vi "available tags menu.vi"(4 "Coords":T2, 5 "parent vi reference":refnum<vi>, 6 "Screen":bool, 8 "error in":errorcluster, 9 "channel to map to":refnum<class "TBM channel.lvclass">, 10 "object ref":T1, 11 "ATM":refnum<user-event>) -> (0 "error out":errorcluster)   [LabVIEW 2013, in "Table Manager.lvlib"]
uses:
  Table Manager.lvlib
  <vilib>/NI/Tag Bus Module Framework/channel/TBM channel.lvclass
  <vilib>/Utility/miscctls.llb/LVPoint32TypeDef.ctl
  <vilib>/NI/DCAF/Tag Editor Core/control module/editor node/channel action event.ctl
  <vilib>/NI/DCAF/Tag Editor Core/control module/editor node/dialog output action.ctl
  <vilib>/NI/Tag Bus/tag/tag descriptor.lvclass
  Table Manager/object ref.ctl
  <vilib>/NI/DCAF/Tag Editor Core/Configuration Editor/Classes/Engine Parent/Engine Parent Editor Node.lvclass
  <vilib>/NI/DCAF/Tag Editor Core/Configuration Editor/Classes/Module editor node/module editor node.lvclass
  <vilib>/NI/DCAF/Tag Editor Core/Configuration Editor/Classes/Engine Parent/read engine configuration.vi
  <vilib>/NI/Module Execution Interface/Engine Configuration/engine configuration.lvclass
  <vilib>/NI/DCAF/Tag Editor Core/control module/editor node/control module editor.lvclass
  Table Manager/Table Manager.lvclass
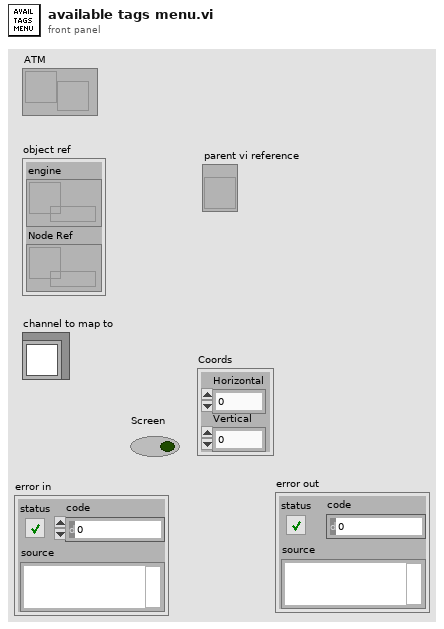
[diagram p1: front panel]
types:
  T1 = typedef "Table Manager.lvlib/Table Manager.lvclass/object ref.ctl" = cluster{"engine":refnum<data-value>, "Node Ref":refnum<data-value>}
  T2 = typedef "LVPoint32TypeDef.ctl" = cluster{"Horizontal":i32, "Vertical":i32}
  T3 = enum32{"Invalid", "Standard", "Closed", "Hidden", "Minimized", "Maximized"}
  T4 = typedef "LVRectTypeDef.ctl" = cluster{"Left":i16, "Top":i16, "Right":i16, "Bottom":i16}
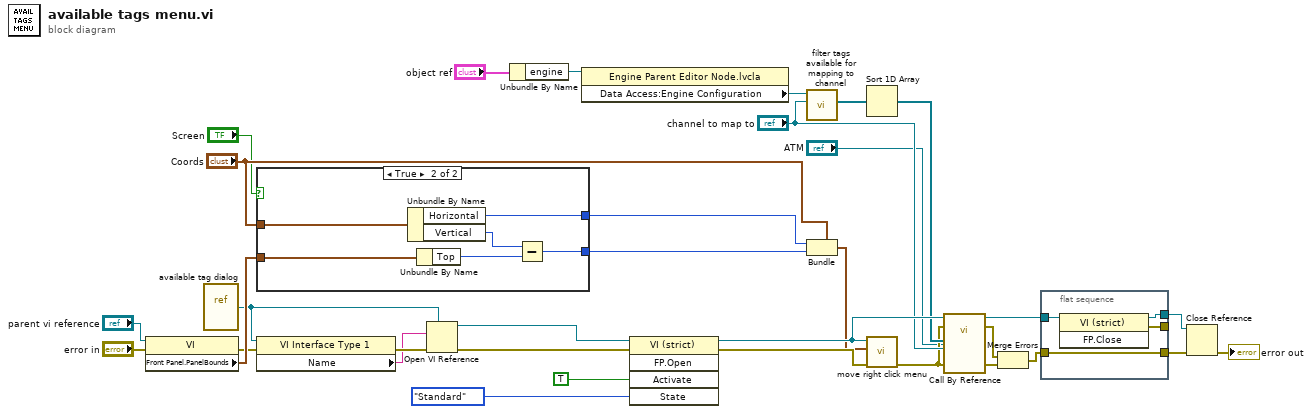
[diagram p0: block diagram]
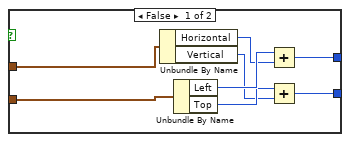
[diagram p2: hidden frame]
diagram:
  n1 = property class="VI"(reference="parent vi reference", error in="error in") -> (error out=w13:errorcluster, "Front Panel.PanelBounds"=w32:T4)  [unwired: 1 out]
  n2 = vi-ref "available tag dialog.vi"() -> (w20:refnum<vi>)
  n3 = case shown="True" "Screen" {
    tunnel: w32 -> [w41 w45]
    tunnel: [w38 w46] -> w31
    tunnel: [w35 w42] -> w30
    tunnel: "Coords" -> [w34 w47]
    frame False {
      n4 = Unbundle By Name(w34) -> ("Horizontal"=w39:i32, "Vertical"=w36:i32)
      n5 = Unbundle By Name(w41) -> ("Left"=w40:i16, "Top"=w37:i16)
      n6 = Add(x=w40, y=w39) -> (x+y=w38:i32)
      n7 = Add(x=w37, y=w36) -> (x+y=w35:i32)
    }
    frame True {
      n8 = Unbundle By Name(w47) -> ("Horizontal"=w46:i32, "Vertical"=w44:i32)
      n9 = Unbundle By Name(w45) -> ("Top"=w43:i16)
      n10 = Subtract(x=w44, y=w43) -> (x-y=w42:i32)
    }
  }
  n11 = property class="VI Interface Type 1"(reference=w20, error in=w13) -> (error out=w27:errorcluster, "Name"=w26:string)  [unwired: 1 out]
  n12 = Open VI Reference(type specifier VI Refnum (for type only)=w20, vi path=w26, error in (no error)=w27) -> (vi reference=w24:refnum<vi>, error out=w25:errorcluster)  [unwired: 3 in]
  n13 = Unbundle By Name("object ref") -> ("engine"=w2:refnum<data-value>)
  n14 = property class="Engine Parent Editor Node.lvcla"(reference=w2) -> ("Data Access:Engine Configuration"=w4:refnum<class "engine configuration.lvclass">)  [unwired: 1 in, 2 out]
  n15 = invoke class="VI (strict)" method="FP.Open"(reference=w24, error in=w25, "Activate"=TRUE ("Activate?"), "State"=T3."Standard") -> (reference out=w19:refnum<vi>, error out=w21:errorcluster)  [unwired: 1 in, 3 out]
  n16 = call <vilib>:"filter tags available for mapping to channel.vi"("channel to map to"="channel to map to", "engine configuration in"=w4) -> ("filtered tags"=w33:refnum<class "tag descriptor.lvclass">[])  [unwired: 8 in, 1 out]
  n17 = Bundle(cluster="Coords", "Horizontal"=w31, "Vertical"=w30) -> (w10:T2)
  n18 = Sort 1D Array(array=w33) -> (sorted array=w11:refnum<class "tag descriptor.lvclass">[])
  n19 = call <vilib>:"move right click menu.vi"("error in"=w21, "Point32"=w10, "VI"=w19) -> ("error out"=w7:errorcluster)  [unwired: 8 in]
  n20 = call-by-ref "?"(reference=w19, error in=w7, "channel action event"="ATM", "error in"=w7, "channel to map to"="channel to map to", "filtered tags"=w11) -> (reference out=w17:refnum<vi>, error out=w18:errorcluster, 0:"error out"=w6:errorcluster)  [unwired: 7 in]
  n21 = Merge Errors(w18, w6) -> (w9:errorcluster)
  n22 = flat-sequence {
    tunnel: w17 -> [w51]
    tunnel: [w50] -> w16
    tunnel: [w49] -> _
    tunnel: w9 -> [w48]
    tunnel: [w48] -> w8
    frame #0 {
      n23 = invoke class="VI (strict)" method="FP.Close"(reference=w51) -> (reference out=w50:refnum<vi>, error out=w49:errorcluster)  [unwired: 2 in, 1 out]
    }
  }
  n24 = Close Reference(reference=w16, error in (no error)=w8) -> (error out=→"error out":errorcluster)
